vi "PCRE-exact match.vi"(6 "quote specials":bool, 9 "regular expression":string="aaa bbb.ccc", 11 "input string":string="aaa bbb.ccc") -> (0 "whole match":string, 3 "exact match":bool=TRUE, 7 "output string":string="aaa bbb.ccc")   [LabVIEW 2015]
uses:
  <vilib>/regexp/Match Regular Expression.xnode
panel:
  out "quoted regular expression":string="aaa bbb.ccc"
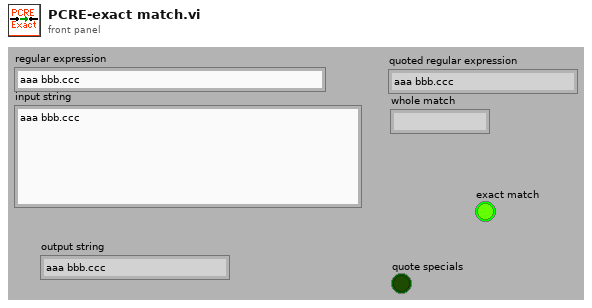
[diagram p1: front panel]
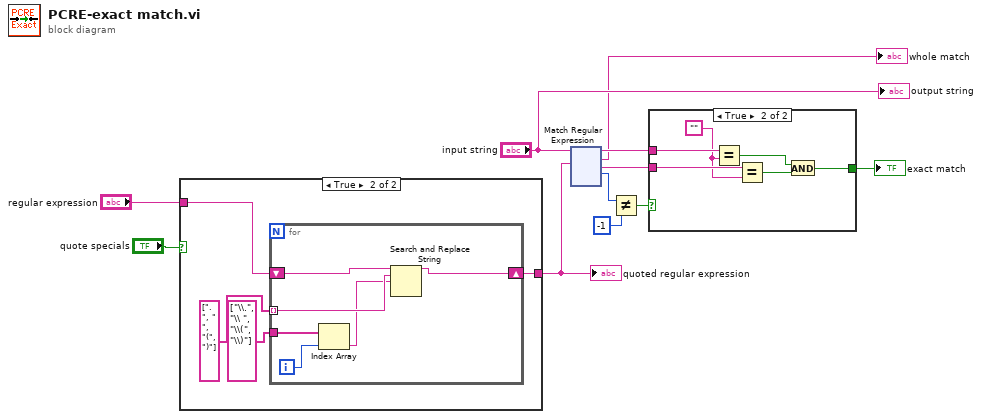
[diagram p0: block diagram]
diagram:
  n1 = case shown="True" "quote specials" {
    tunnel: [w12 w15] -> w3
    tunnel: "regular expression" -> [w12 w14]
    frame False {
    }
    frame True {
      n2 = for {
        tunnel: string[] [".", " ", "(", ")"] -> [w21] mode=indexing
        shift-right: [w20] -> w15
        shift-left: w14 -> [w22]
        tunnel: string[] ["\\.", "\\ ", "\\(", "\\)"] -> [w18]
        i -> [w19]
        n3 = Index Array(array=w18, index=w19) -> (element=w17:string)
        n4 = Search and Replace String(input string=w22, search string=w21, replace string=w17) -> (result string=w20:string)  [unwired: 5 in, 3 out]
      }
    }
  }
  "quoted regular expression" <- w3
  n5 = xnode "Match Regular Expression"("input string"="input string", "regular expression"=w3) -> ("before match"=w8:string, "whole match"=→"whole match":string, "after match"=w11:string, "offset past match"=w10:i32)  [unwired: 4 in, 1 out]
  n6 = Not Equal?(x=w10, y=-1) -> (x != y?=w7:bool)
  n7 = case shown="True" w7 {
    selector: w7 -> [w23 _]
    tunnel: w11 -> [_ w29]
    tunnel: w8 -> [_ w25]
    tunnel: [w23 w26] -> w6
    frame False {
    }
    frame True {
      w24 = ""
      n8 = Equal?(x=w25, y=w24) -> (x = y?=w27:bool)
      n9 = Equal?(x=w29, y=w24) -> (x = y?=w28:bool)
      n10 = And(x=w27, y=w28) -> (x .and. y?=w26:bool)
    }
  }
  "exact match" <- w6
  "output string" <- "input string"
